vi "Control Test.vi"() -> ()   [LabVIEW 2015, in "Peltier.lvclass"]
uses:
  Peltier.lvclass
  Typedefs/Peltier Temperature Sensors.ctl
panel:
  out "Set Point":dbl
  out "Kd":u8
  out "Ki":u8
  out "Kp":u8
  out "After":dbl[](array[numeric])
  out "Before":dbl[](array[numeric])
  in  "stop":bool
  out "error out":errorcluster
  out "Ready?":bool
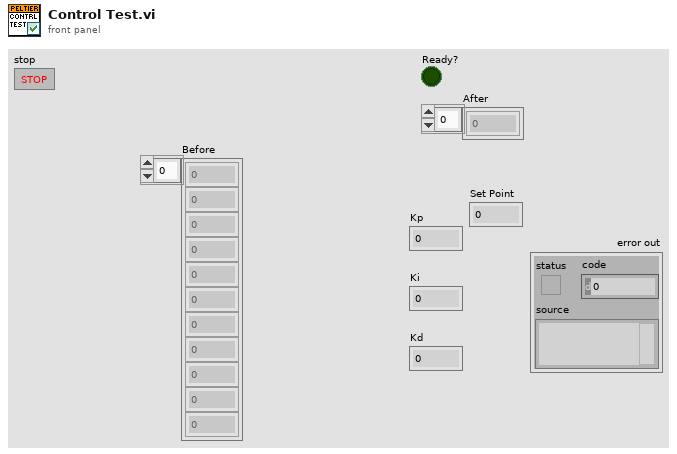
[diagram p1: front panel]
types:
  T1 = typedef "Peltier.lvclass/Peltier Temperature Sensors.ctl" = u16
  T2 = typedef "Peltier.lvclass/Session Handle.ctl" = refnum<data-value>
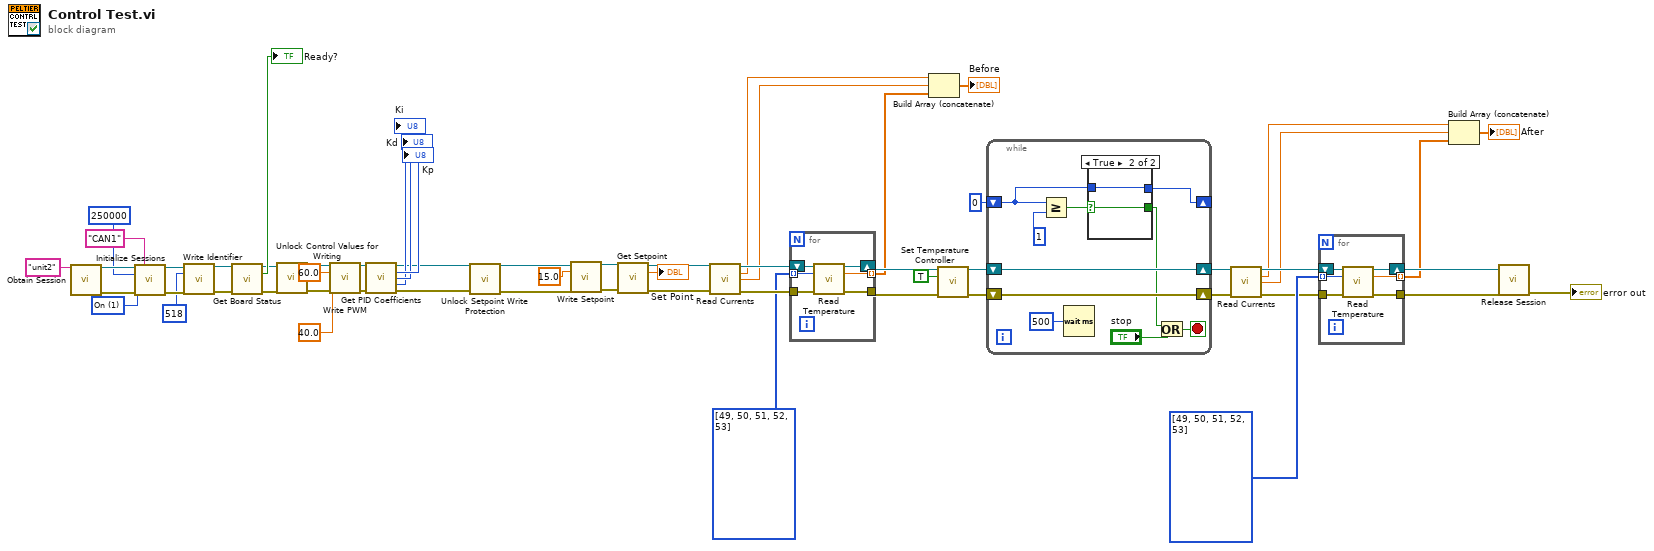
[diagram p0: block diagram]
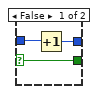
[diagram p2: hidden frame]
diagram:
  w40 = T1[] [49, 50, 51, 52, 53] items=["PTS1"=49, "PTS2"=50, "PTS3"=51, "PTS4"=52, "PTS5"=53, "PTS6"=54]
  w44 = T1[] [49, 50, 51, 52, 53] items=["PTS1"=49, "PTS2"=50, "PTS3"=51, "PTS4"=52, "PTS5"=53, "PTS6"=54]
  w54 = u32 1 items=["Off", "On"] ("Termination")
  n1 = call "Obtain Session.vi"("Session  Name ()"="unit2") -> ("Session Handle"=w57:T2, "error out"=w56:errorcluster)  [unwired: 13 in]
  n2 = call "Initialize Sessions.vi"("Session Handle"=w57, "CAN Interface"="CAN1", "Baud Rate"=u32 250000, "Termination"=w54, "error in (no error)"=w56) -> ("Session Handle Out"=w53:T2, "error out"=w52:errorcluster)  [unwired: 9 in]
  n3 = call "Write Identifier.vi"("Session Handle In"=w53, "identifier"=u16 518, "error in (no error)"=w52) -> ("Session Handle Out"=w50:T2, "error out"=w49:errorcluster)  [unwired: 11 in]
  n4 = call "Get Board Status.vi"("Session Handle"=w50, "error in (no error)"=w49) -> ("Session Handle Out"=w27:T2, "Ready?"=→"Ready?":bool, "error out"=w26:errorcluster)  [unwired: 11 in]
  n5 = call "Unlock Control Values for Writing.vi"("Session Handle"=w27, "error in (no error)"=w26) -> ("Session Handle Out"=w25:T2, "error out"=w24:errorcluster)  [unwired: 12 in]
  n6 = call "Write PWM.vi"("Session Handle"=w25, "Max PWM"=60.0, "Min PWM"=40.0, "error in (no error)"=w24) -> ("Session Handle Out"=w16:T2, "error out"=w15:errorcluster)  [unwired: 10 in]
  n7 = call "Get PID Coefficients.vi"("Session Handle"=w16, "error in (no error)"=w15) -> ("Session Handle Out"=w5:T2, "Kp"=→"Kp":u8, "Ki"=→"Ki":u8, "Kd"=→"Kd":u8, "error out"=w3:errorcluster)  [unwired: 9 in]
  n8 = call "Unlock Setpoint Write Protection.vi"("Session Handle"=w5, "error in (no error)"=w3) -> ("Session Handle Out"=w4:T2, "error out"=w2:errorcluster)  [unwired: 12 in]
  n9 = call "Write Setpoint.vi"("Session Handle"=w4, "Setpoint"=15.0, "error in (no error)"=w2) -> ("Session Handle Out"=w7:T2, "error out"=w6:errorcluster)  [unwired: 11 in]
  n10 = call "Get Setpoint.vi"("Session Handle"=w7, "error in (no error)"=w6) -> ("Session Handle Out"=w10:T2, "Set Point"=→"Set Point":dbl, "error out"=w11:errorcluster)  [unwired: 11 in]
  n11 = call "Read Currents.vi"("Session Handle"=w10, "error in (no error)"=w11) -> ("Session Handle Out"=w46:T2, "Side 1 Current"=w35:dbl, "Side 2 Current"=w34:dbl, "error out"=w45:errorcluster)  [unwired: 10 in]
  n12 = for {
    tunnel: w45 -> [w63]
    shift-right: [w60] -> w42
    shift-left: w46 -> [w64]
    tunnel: [w62] -> w43
    tunnel: w44 -> [w61] mode=indexing
    tunnel: [w59] -> w33 mode=indexing
    n13 = call "Read Temperature.vi"("Session Handle"=w64, "Pelt Temp Sensors"=w61, "error in (no error)"=w63) -> ("Session Handle Out"=w60:T2, "Temperature"=w59:dbl, "error out"=w62:errorcluster)  [unwired: 10 in]
  }
  n14 = Build Array (concatenate)(w35, w34, w33) -> (→"Before":dbl[])
  n15 = call "Set Temperature Controller.vi"("Session Handle"=w42, "On?"=TRUE, "error in (no error)"=w43) -> ("Session Handle Out"=w32:T2, "error out"=w31:errorcluster)  [unwired: 11 in]
  n16 = while {
    shift-right: [w74] -> w29
    shift-left: w32 -> [w74]
    shift-right: [w73] -> w28
    shift-left: w31 -> [w73]
    shift-right: [w66] -> _
    shift-left: 0 -> [w67]
    stop <- w65 stop-if-true
    n17 = Greater Or Equal?(x=w67, y=1) -> (x >= y?=w70:bool)
    n18 = Wait (ms)(milliseconds to wait=u32 500) -> ()  [unwired: 1 out]
    n19 = case shown="True" w70 {
      selector: w70 -> [w75 w79]
      tunnel: [w75 w79] -> w68
      tunnel: w67 -> [w77 w78]
      tunnel: [w76 w78] -> w66
      frame False {
        n20 = Increment(x=w77) -> (x+1=w76:i32)
      }
      frame True {
      }
    }
    n21 = Or(x=w68, y="stop") -> (x .or. y?=w65:bool)
  }
  n22 = call "Read Currents.vi"("Session Handle"=w29, "error in (no error)"=w28) -> ("Session Handle Out"=w38:T2, "Side 1 Current"=w20:dbl, "Side 2 Current"=w19:dbl, "error out"=w39:errorcluster)  [unwired: 10 in]
  n23 = for {
    tunnel: w39 -> [w84]
    shift-right: [w81] -> w36
    shift-left: w38 -> [w85]
    tunnel: [w83] -> w37
    tunnel: w40 -> [w82] mode=indexing
    tunnel: [w80] -> w18 mode=indexing
    n24 = call "Read Temperature.vi"("Session Handle"=w85, "Pelt Temp Sensors"=w82, "error in (no error)"=w84) -> ("Session Handle Out"=w81:T2, "Temperature"=w80:dbl, "error out"=w83:errorcluster)  [unwired: 10 in]
  }
  n25 = Build Array (concatenate)(w20, w19, w18) -> (→"After":dbl[])
  n26 = call "Release Session.vi"("Session Handle"=w36, "error in (no error)"=w37) -> ("error out"=→"error out":errorcluster)  [unwired: 13 in]
